vi "implementEcho_Init.vi"(0 "object in":refnum<class "implementEcho.lvclass">, 5 "error in (no error)":errorcluster) -> (14 "object out":refnum<class "implementEcho.lvclass">, 19 "error out":errorcluster)   [LabVIEW 2015, in "UserManagement.lvlib" / "implementEcho.lvclass"]
uses:
  implementEcho.lvclass
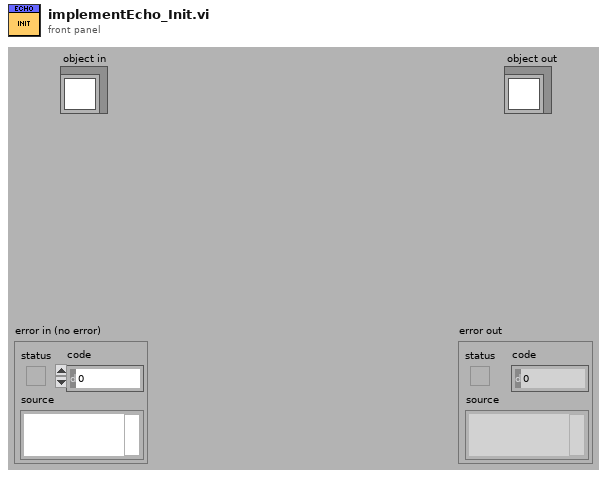
[diagram p1: front panel]
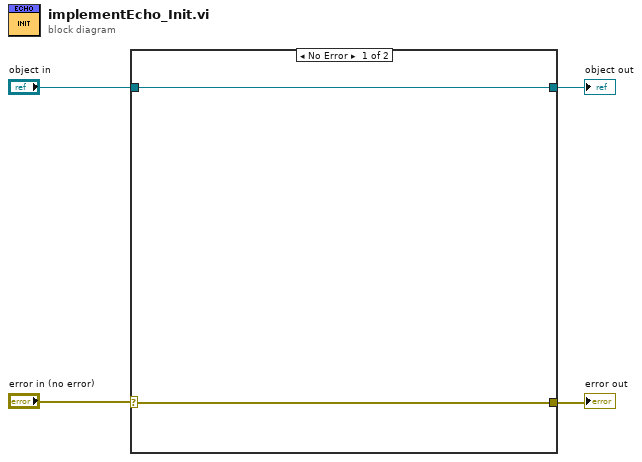
[diagram p0: block diagram]
diagram:
  n1 = case shown="No Error" "error in (no error)" {
    selector: "error in (no error)" -> [w5 w7]
    tunnel: "object in" -> [w6 w8]
    tunnel: [w6 w8] -> w3
    tunnel: [w5 w7] -> w1
    frame No Error {
    }
    frame Error {
    }
  }
  "object out" <- w3
  "error out" <- w1
